vi "mes参数配置.vi"() -> ()   [LabVIEW 2015]
uses:
  Global.vi
panel:
  in  "取消":bool
  in  "确定":bool
  in  "MES参数":T1
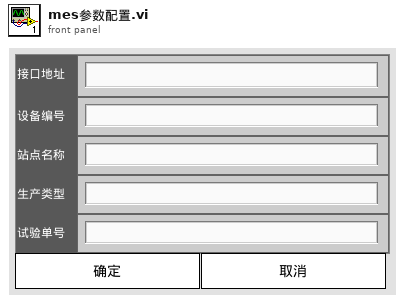
[diagram p1: front panel]
types:
  T1 = cluster{"接口地址":string, "设备编号":string, "站点名称":string, "生产类型":string, "试验单号":string}
  T2 = cluster{"接口地址(URL)":string, "设备编号(equipNum)":string, "站点名称(siteCode)":string, "生产类型(productType)":string, "试验单号(testOrderNum)":string}
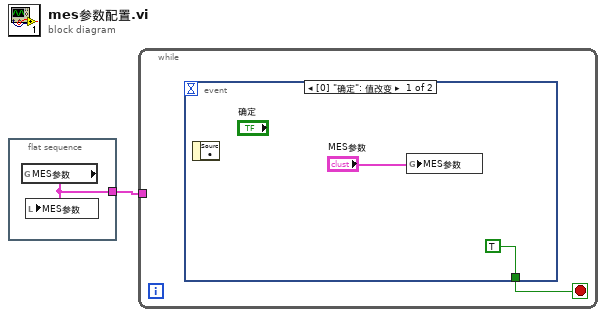
[diagram p0: block diagram]
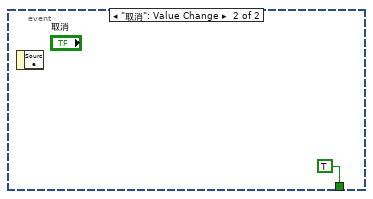
[diagram p2: hidden frame]
diagram:
  n1 = flat-sequence {
    tunnel: [w2] -> w1
    frame #0 {
      n2 = global read "Global.vi" "MES参数"() -> (w2:T2)
      n3 = local write "MES参数"(w2) -> ()
    }
  }
  n4 = while {
    tunnel: w1 -> [_]
    stop <- w3 stop-if-true
    n5 = event shown="[0] \"确定\": 值改变" {
      selector: _ -> [_ _]
      dyn-events: _ -> [_ _]
      timeout: _ -> [_ _]
      tunnel: [TRUE TRUE] -> w3
      event "确定": Value Change {
        n6 = event-data() -> ()  [unwired: 1 in, 1 out]
        n7 = global write "Global.vi" "MES参数"("MES参数") -> ()
      }
      event "取消": Value Change {
        n8 = event-data() -> ()  [unwired: 1 in, 1 out]
      }
    }
  }
